vi "APC_9049_LoadWarningConfig.vi"(2 "CylinderDiagnosticsCluster":T1={"samples for running IMEP std"=100, "MaxDevFromExpectedIMEPError [bar]"=2.0, "MaxDevFromExpectedIMEPWarning [bar]"=2.0, "MaxDevFromAvgError [bar]"=2.0, "MaxDevFromSelfAvgWarning [bar]"=2.0, "MaxDevFromSelfAvgError [bar]"=2.0, "MaxDevFromAvgWarning [bar]"=2.0, "MaxIMEPstdWarning [bar]"=0.5, "MaxIMEPstdError [bar]"=0.5, "MAPOmaxError [bar/CAD]"=1.0, "MAPOmaxWarning [bar/CAD]"=1.0, "CA50maxError [CADATDC]"=15.0, "CA50maxWarning [CADATDC]"=15.0, "MaxPCylMaxError [bar]"=120.0, "MaxPCylMaxWarning [bar]"=120.0}, 3 "Load?":bool=TRUE) -> (0 "CylinderDiagnosticsCluster 2":T1={"samples for running IMEP std"=100, "MaxDevFromExpectedIMEPError [bar]"=2.0, "MaxDevFromExpectedIMEPWarning [bar]"=2.0, "MaxDevFromAvgError [bar]"=2.0, "MaxDevFromSelfAvgWarning [bar]"=2.0, "MaxDevFromSelfAvgError [bar]"=2.0, "MaxDevFromAvgWarning [bar]"=2.0, "MaxIMEPstdWarning [bar]"=0.5, "MaxIMEPstdError [bar]"=0.5, "MAPOmaxError [bar/CAD]"=1.0, "MAPOmaxWarning [bar/CAD]"=1.0, "CA50maxError [CADATDC]"=15.0, "CA50maxWarning [CADATDC]"=15.0, "MaxPCylMaxError [bar]"=120.0, "MaxPCylMaxWarning [bar]"=120.0})   [LabVIEW 2020]
uses:
  controls/APC_CylDaignosticsCluster.ctl
  <vilib>/Utility/xml.llb/Write to XML File(string).vi
  <vilib>/Utility/xml.llb/Read From XML File(string).vi
panel:
  out "error out":errorcluster
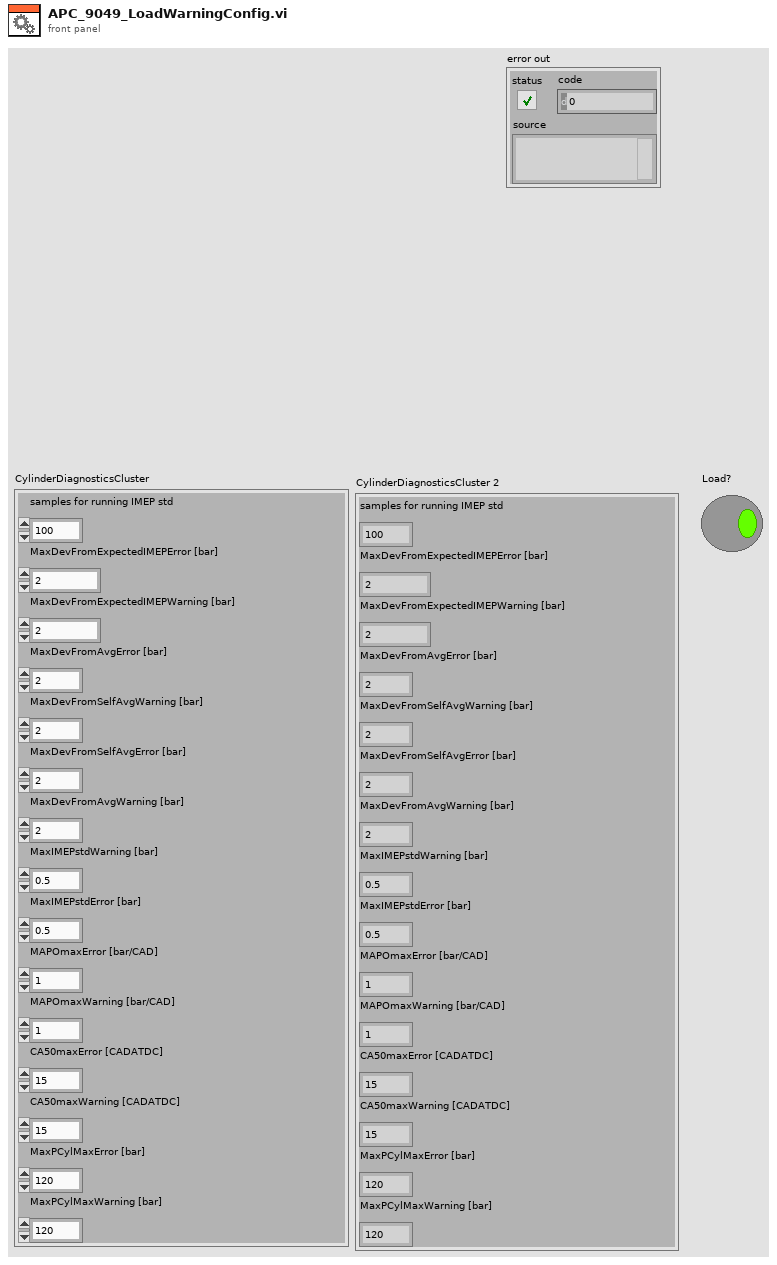
[diagram p1: front panel]
types:
  T1 = typedef "APC_CylDaignosticsCluster.ctl" = cluster{"samples for running IMEP std":i32, "MaxDevFromExpectedIMEPError [bar]":dbl, "MaxDevFromExpectedIMEPWarning [bar]":dbl, "MaxDevFromAvgError [bar]":dbl, "MaxDevFromSelfAvgWarning [bar]":dbl, "MaxDevFromSelfAvgError [bar]":dbl, "MaxDevFromAvgWarning [bar]":dbl, "MaxIMEPstdWarning [bar]":dbl, "MaxIMEPstdError [bar]":dbl, "MAPOmaxError [bar/CAD]":dbl, "MAPOmaxWarning [bar/CAD]":dbl, "CA50maxError [CADATDC]":dbl, "CA50maxWarning [CADATDC]":dbl, "MaxPCylMaxError [bar]":dbl, "MaxPCylMaxWarning [bar]":dbl}
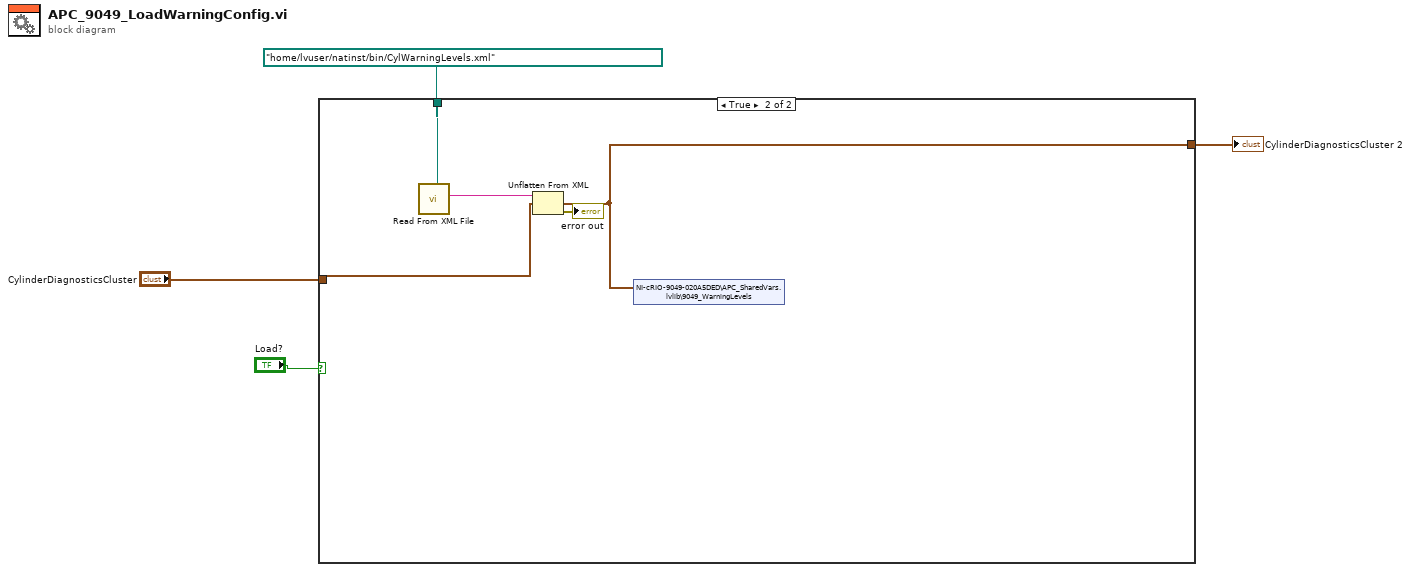
[diagram p0: block diagram]
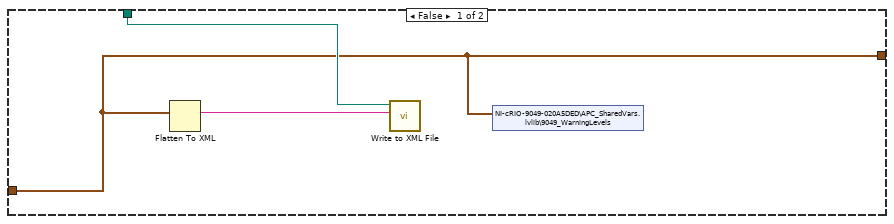
[diagram p2: hidden frame]
diagram:
  n1 = case shown="True" "Load?" {
    tunnel: "CylinderDiagnosticsCluster" -> [w5 w11]
    tunnel: path "/home/lvuser/natinst/bin/CylWarningLevels.xml" ("XML File Path") -> [w6 w10]
    tunnel: [w5 w9] -> w1
    frame False {
      n2 = Flatten To XML(6:w5) -> (2:w7:string)
      n3 = call-poly <vilib>:"Write to XML File.vi"("XML Input"=w7, "XML File Path"=w6) -> ()  [unwired: 7 in, 3 out]
      n4 = shared-variable "NI-cRIO-9049-020A5DED\\APC_SharedVars.lvlib\\9049_WarningLevels"(w5) -> ()  [unwired: 1 in, 1 out]
    }
    frame True {
      n5 = call-poly <vilib>:"Read From XML File.vi"("XML File Path"=w10) -> ("XML Elements"=w12:string)  [unwired: 8 in, 2 out]
      n6 = Unflatten From XML(xml string=w12, type=w11) -> (value=w9:T1, error out=→"error out":errorcluster)  [unwired: 1 in]
      n7 = shared-variable "NI-cRIO-9049-020A5DED\\APC_SharedVars.lvlib\\9049_WarningLevels"(w9) -> ()  [unwired: 1 in, 1 out]
    }
  }
  "CylinderDiagnosticsCluster 2" <- w1
